vi "Test VI 02.vi"(8 "Error In":errorcluster) -> (0 "Error Out":errorcluster)   [LabVIEW 2013, in "library-under-test.lvlib"]
uses:
  library-under-test.lvlib
  classes/Assert/Assert Equal Value_Variant.vi
  classes/Test/Test.lvclass
  classes/Assert/Assert.lvclass
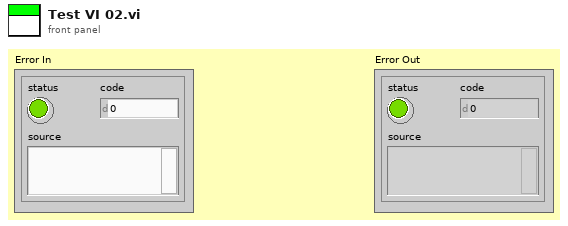
[diagram p1: front panel]
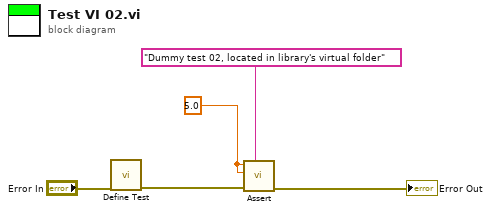
[diagram p0: block diagram]
diagram:
  w2 = 5.0
  n1 = call "Define Test.vi"("error in (no error)"="Error In") -> ("error out"=w4:errorcluster)  [unwired: 10 in]
  n2 = call-poly "Assert.vi"("Label"="Dummy test 02, located in library's virtual folder", "error in (no error)"=w4, "Y"=w2, "X"=w2) -> ("error out"=→"Error Out":errorcluster)  [unwired: 7 in]
